vi "shift_left_polynomial.vi"(1 "Polynomial":u8[](array[numeric])) -> (0 "Polynomial * 2":u8[](array[numeric]))   [LabVIEW 2022 SP3]
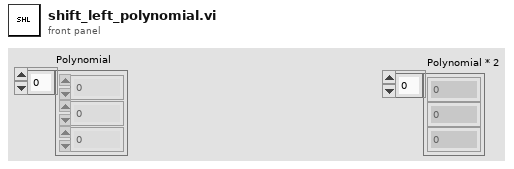
[diagram p1: front panel]
types:
  T1 = cluster{"Polynomial[0]":u8, "Polynomial[1]":u8, "Polynomial[2]":u8}
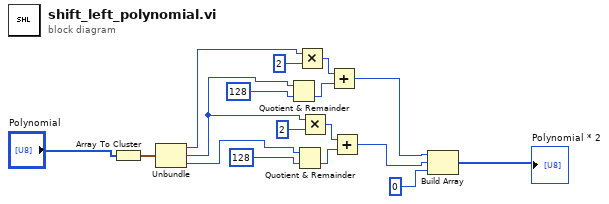
[diagram p0: block diagram]
diagram:
  n1 = Array To Cluster(array="Polynomial") -> (cluster=w17:T1)
  n2 = Unbundle(w17) -> ("Polynomial[0]"=w7:u8, "Polynomial[1]"=w3:u8, "Polynomial[2]"=w5:u8)
  n3 = Quotient & Remainder(x=w3, y=u8 128) -> (floor(x/y)=w1:u8)  [unwired: 1 out]
  n4 = Quotient & Remainder(x=w5, y=u8 128) -> (floor(x/y)=w6:u8)  [unwired: 1 out]
  n5 = Multiply(x=w7, y=u8 2) -> (x*y=w15:u8)
  n6 = Multiply(x=w3, y=u8 2) -> (x*y=w13:u8)
  n7 = Add(x=w15, y=w1) -> (x+y=w8:u8)
  n8 = Add(x=w13, y=w6) -> (x+y=w9:u8)
  n9 = Build Array(w8, w9, u8 0 ("element")) -> (→"Polynomial * 2":u8[])
